vi "K2450 Set Voltage and Wait.vi"(8 "Error In":errorcluster, 9 "Wait After Setting":dbl=3.0 format="%<%M:%S>t", 10 "Voltage":dbl, 11 "VISA resource name":refnum<visa-resource-name>) -> (0 "Error Out":errorcluster, 3 "VISA resource name Out":refnum<visa-resource-name>)   [LabVIEW 2020]
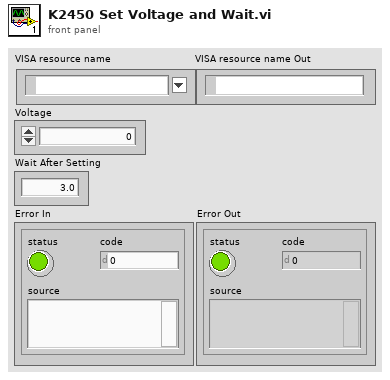
[diagram p1: front panel]
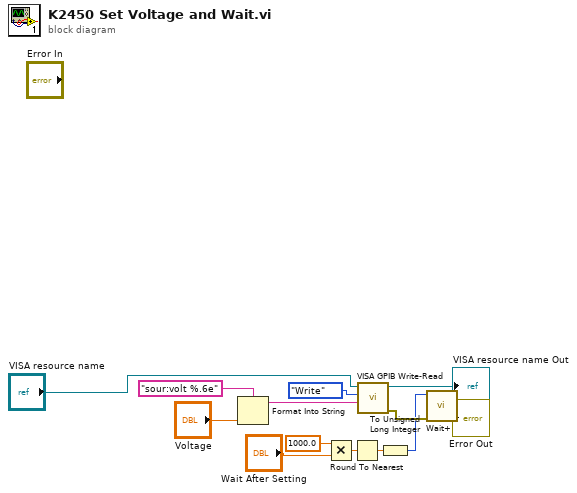
[diagram p0: block diagram]
diagram:
  n1 = Format Into String(format string="sour:volt %.6e", "Voltage") -> (resulting string=w1:string)  [unwired: 2 in, 1 out]
  n2 = Multiply(x=1000.0, y="Wait After Setting") -> (x*y=w9:dbl)
  n3 = Round To Nearest(number=w9) -> (nearest integer value=w10:dbl)
  n4 = call "VISA GPIB Write-Read.vi"("Command"=w1, "Action"=enum16{"Write", "Read", "Write & Read"}."Write", "VISA resource name"="VISA resource name") -> ("error out"=w13:errorcluster, "dup VISA Session"=→"VISA resource name Out":refnum<visa-resource-name>)  [unwired: 5 in, 2 out]
  n5 = To Unsigned Long Integer(number=w10) -> (unsigned 32bit integer=w7:u32)
  n6 = call "Wait+.vi"("Error In"=w13, "milliseconds to wait"=w7) -> ("Error Out"=→"Error Out":errorcluster)  [unwired: 4 in, 1 out]
